vi "TrapProfState_Equals.vi"(9 "TRAPEZOID_PROFILE_STATE 2":T1 {"Velocity" format="%16_6e"; "Position" format="%16_6e"}, 11 "TRAPEZOID_PROFILE_STATE":T1 {"Velocity" format="%16_6e"; "Position" format="%16_6e"}) -> (3 "Equal":bool)   [LabVIEW 2019, in "Trajectory_Library.lvlib"]
doc: "Compares the values of two Trapezoid Profile States. If both are EXACTLY equal, True is returned.\n\nInputs:\n - Trapezoid_Profile_state -- The first state to compare\n - Trapezoid_Profile_state_2 -- The second state to comapre\n\nOutputs:\n - Equal -- True if both states are identical."
uses:
  Trajectory_Library.lvlib
  TRAPEZOID_PROFILE_STATE.ctl
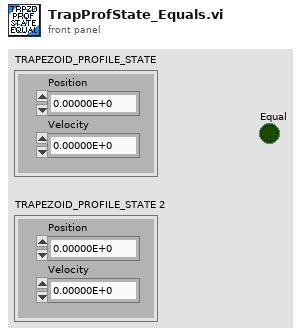
[diagram p1: front panel]
types:
  T1 = typedef "Trajectory_Library.lvlib/TRAPEZOID_PROFILE_STATE.ctl" = cluster{"Position":dbl, "Velocity":dbl}
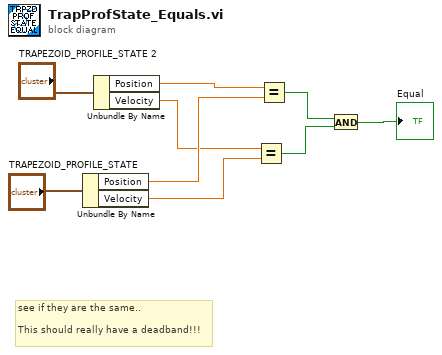
[diagram p0: block diagram]
diagram:
  # "see if they are the same..\n\nThis should really have a deadband!!!"
  n1 = Unbundle By Name("TRAPEZOID_PROFILE_STATE") -> ("Position"=w6:dbl, "Velocity"=w4:dbl)
  n2 = Unbundle By Name("TRAPEZOID_PROFILE_STATE 2") -> ("Position"=w7:dbl, "Velocity"=w5:dbl)
  n3 = Equal?(x=w5, y=w4) -> (x = y?=w2:bool)
  n4 = Equal?(x=w7, y=w6) -> (x = y?=w3:bool)
  n5 = And(x=w3, y=w2) -> (x .and. y?=→"Equal":bool)
